vi "Extract Data2D.vi"(8 "error in (no error)":errorcluster, 10 "Data2D in":refnum<class "Data2D.lvclass">, 11 "ImagingExtractor in":refnum<class "ImagingExtractor.lvclass">) -> (0 "error out":errorcluster, 3 "ImagingExtractor out":refnum<class "ImagingExtractor.lvclass">)   [LabVIEW 2014, in "ImagingExtractor.lvclass"]
uses:
  ImagingExtractor.lvclass
  Framework/Model/Data/Data2D/Data2D.lvclass
  Framework/Interfaces/Observable Actor/Observable Actor.lvclass
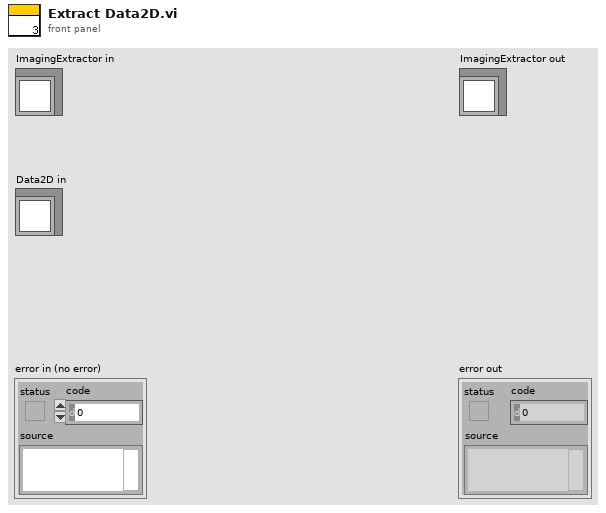
[diagram p1: front panel]
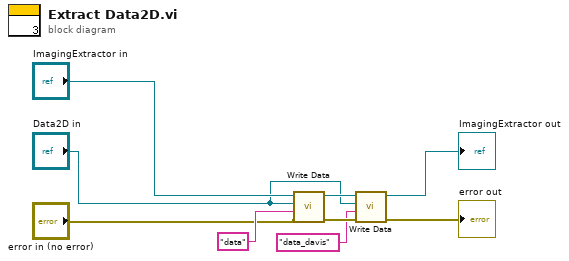
[diagram p0: block diagram]
diagram:
  n1 = call "Write Data.vi"("error in (no error)"="error in (no error)", "Name"="data", "Data"="Data2D in", "Observable Actor in"="ImagingExtractor in") -> ("error out"=w4:errorcluster, "Observable Actor out"=w6:refnum<class "ImagingExtractor.lvclass">)  [unwired: 6 in]
  n2 = call "Write Data.vi"("error in (no error)"=w4, "Name"="data_davis", "Data"="Data2D in", "Observable Actor in"=w6) -> ("error out"=→"error out":errorcluster, "Observable Actor out"=→"ImagingExtractor out":refnum<class "ImagingExtractor.lvclass">)  [unwired: 6 in]
